vi "IssueRunID.vi"(1 "data storage path":path) -> (0 "Run ID":string)   [LabVIEW 2021]
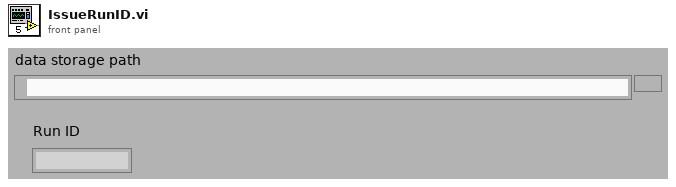
[diagram p1: front panel]
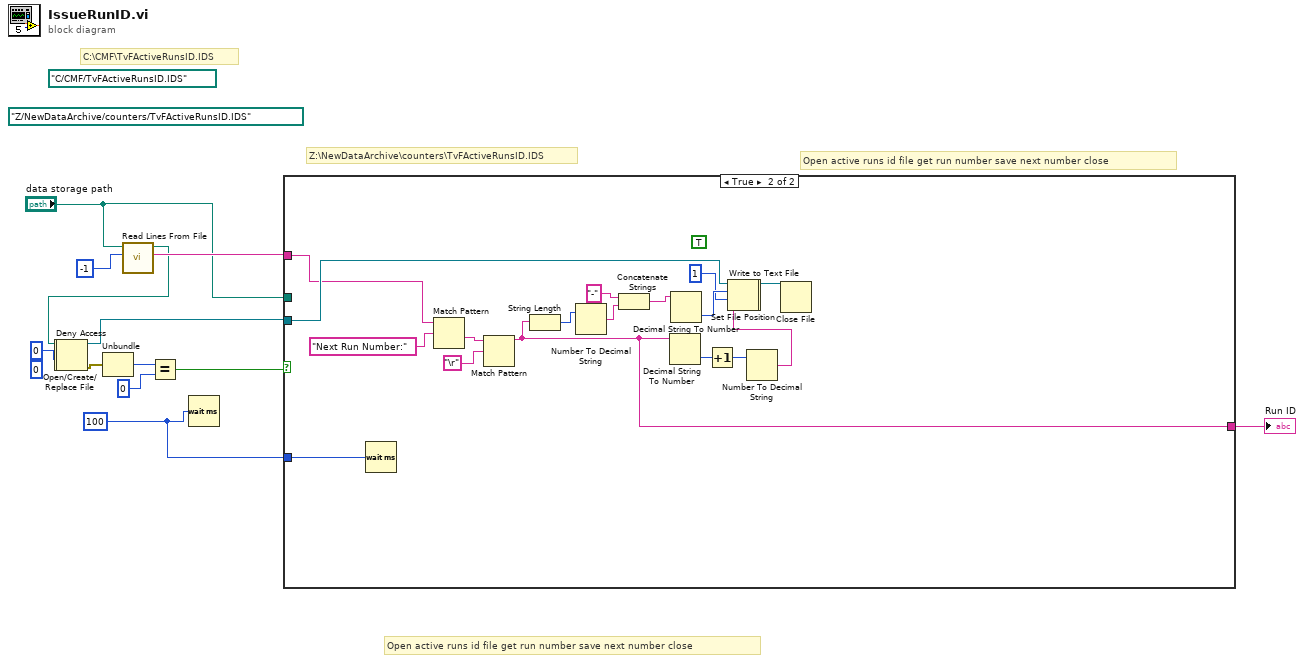
[diagram p0: block diagram]
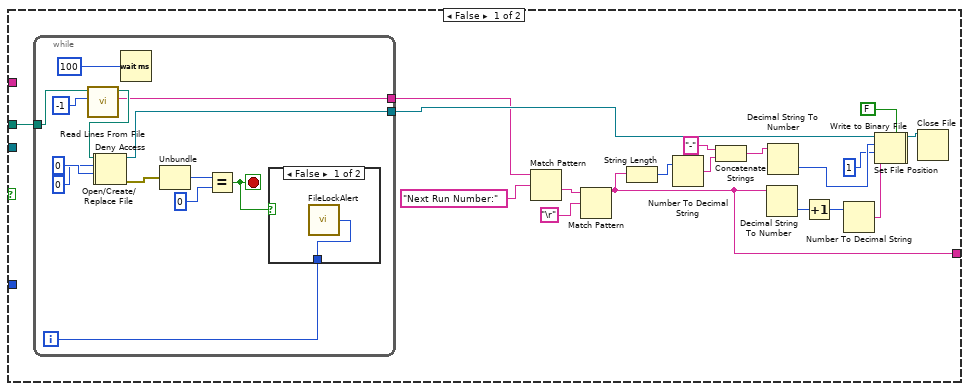
[diagram p2: hidden frame]
diagram:
  (unwired) path "Z:/NewDataArchive/counters/TvFActiveRunsID.IDS"
  (unwired) path "C:/CMF/TvFActiveRunsID.IDS"
  w4 = 100
  # "C:\\CMF\\TvFActiveRunsID.IDS"
  # "Open active runs id file get run number save next number close"
  # "Z:\\NewDataArchive\\counters\\TvFActiveRunsID.IDS"
  # "Open active runs id file get run number save next number close"
  n1 = call <vilib>:"Read Lines From File.vi"("file path (dialog if empty)"="data storage path", "number of lines (all:-1)"=-1) -> ("new file path (Not A Path if cancelled)"=w6:path, "line string"=w7:string)  [unwired: 4 in, 2 out]
  n2 = Open/Create/Replace File(file path (use dialog)=w6, access (0:read/write)=0) -> (refnum out=w1:refnum<file>, error out=w2:errorcluster)  [unwired: 4 in, 1 out]
  n3 = Deny Access(4:w2, 6:0, 7:w1) -> (0:w12:errorcluster, 3:w15:refnum<file>)
  n4 = Unbundle(w12) -> ("code"=w11:i32)  [unwired: 2 out]
  n5 = Equal?(x=w11, y=0) -> (x = y?=w9:bool)
  n6 = Wait (ms)(milliseconds to wait=w4) -> ()  [unwired: 1 out]
  n7 = case shown="True" w9 {
    tunnel: w15 -> [_ w59]
    tunnel: [w21 w56] -> w5
    tunnel: w7 -> [_ w55]
    tunnel: "data storage path" -> [w20 _]
    tunnel: w4 -> [_ w54]
    frame False {
      n8 = while {
        tunnel: [w45] -> w23
        tunnel: w20 -> [w40]
        tunnel: [w38] -> w19
        i -> [w42]
        stop <- w43 stop-if-true
        n9 = call <vilib>:"Read Lines From File.vi"("file path (dialog if empty)"=w40, "number of lines (all:-1)"=-1) -> ("new file path (Not A Path if cancelled)"=w39:path, "line string"=w38:string)  [unwired: 4 in, 2 out]
        n10 = Open/Create/Replace File(file path (use dialog)=w39, access (0:read/write)=0) -> (refnum out=w36:refnum<file>, error out=w37:errorcluster)  [unwired: 4 in, 1 out]
        n11 = Deny Access(4:w37, 6:0, 7:w36) -> (0:w48:errorcluster, 3:w45:refnum<file>)
        n12 = Wait (ms)(milliseconds to wait=100) -> ()  [unwired: 1 out]
        n13 = Unbundle(w48) -> ("code"=w47:i32)  [unwired: 2 out]
        n14 = Equal?(x=w47, y=0) -> (x = y?=w43:bool)
        n15 = case shown="False" w43 {
          tunnel: w42 -> [w51 _]
          frame False {
            n16 = call "FileLockAlert.vi"("Retry Cycle Count"=w51) -> ()
          }
          frame True {
          }
        }
      }
      n17 = Match Pattern(string=w19, regular expression="Next Run Number:") -> (after substring=w30:string)  [unwired: 1 in, 3 out]
      n18 = Match Pattern(string=w30, regular expression="\r") -> (before substring=w21:string)  [unwired: 1 in, 3 out]
      n19 = String Length(string=w21) -> (length=w31:i32)
      n20 = Number To Decimal String(number=w31) -> (decimal integer string=w32:string)  [unwired: 1 in]
      n21 = Concatenate Strings("-", w32) -> (w34:string)
      n22 = Decimal String To Number(string=w21) -> (number=w28:i32)  [unwired: 2 in, 1 out]
      n23 = Decimal String To Number(string=w34) -> (number=w35:i32)  [unwired: 2 in, 1 out]
      n24 = Increment(x=w28) -> (x+1=w27:i32)
      n25 = Number To Decimal String(number=w27) -> (decimal integer string=w22:string)  [unwired: 1 in]
      n26 = Set File Position(offset (in bytes) (0)=w35, refnum=w23, from (0:start)=1) -> (refnum out=w18:refnum<file>, error out=w17:errorcluster)  [unwired: 1 in]
      n27 = Write to Binary File(file (use dialog)=w18, data=w22, error in=w17, 5:FALSE ("prepend array or string size? (T)")) -> (refnum out=w24:refnum<file>)  [unwired: 2 in, 2 out]
      n28 = Close File(refnum=w24) -> ()  [unwired: 1 in, 2 out]
    }
    frame True {
      (unwired) TRUE
      n29 = Wait (ms)(milliseconds to wait=w54) -> ()  [unwired: 1 out]
      n30 = Match Pattern(string=w55, regular expression="Next Run Number:") -> (after substring=w65:string)  [unwired: 1 in, 3 out]
      n31 = Match Pattern(string=w65, regular expression="\r") -> (before substring=w56:string)  [unwired: 1 in, 3 out]
      n32 = String Length(string=w56) -> (length=w66:i32)
      n33 = Number To Decimal String(number=w66) -> (decimal integer string=w67:string)  [unwired: 1 in]
      n34 = Concatenate Strings("-", w67) -> (w69:string)
      n35 = Decimal String To Number(string=w56) -> (number=w63:i32)  [unwired: 2 in, 1 out]
      n36 = Decimal String To Number(string=w69) -> (number=w70:i32)  [unwired: 2 in, 1 out]
      n37 = Increment(x=w63) -> (x+1=w62:i32)
      n38 = Set File Position(offset (in bytes) (0)=w70, refnum=w59, from (0:start)=1) -> (refnum out=w53:refnum<file>, error out=w52:errorcluster)  [unwired: 1 in]
      n39 = Number To Decimal String(number=w62) -> (decimal integer string=w57:string)  [unwired: 1 in]
      n40 = Write to Text File(file (use dialog)=w53, text=w57, error in=w52) -> (refnum out=w58:refnum<file>)  [unwired: 1 in, 2 out]
      n41 = Close File(refnum=w58) -> ()  [unwired: 1 in, 2 out]
    }
  }
  "Run ID" <- w5
